vi "SetBaseCluster.vi"(7 "Actor":refnum<class "Actor.lvclass">, 11 "BaseCluster":T1) -> (5 "Actor":refnum<class "Actor.lvclass">)   [LabVIEW 2020, in "_Template.lvlib" / "{{Actor}}.lvlib" / "Actor.lvclass"]
uses:
  Actor.lvclass
  Actor.lvclass/Actor.ctl
  jettl/jettl/Actor/Actor.lvclass
  jettl/jettl/LifecycleEnum.ctl
  jettl/jettl/jettl.lvlib
  jettl/jettl/Message/Message.lvclass
  jettl/jettl/MessageSet.ctl
  jettl/jettl/MessagesCluster.ctl
  jettl/jettl/MessageCluster.ctl
  jettl/jettl/ActorTypeEnum.ctl
  jettl/jettl/ActorCluster.ctl
  jettl/jettl/ComponentActorClusterMap.ctl
  jettl/jettl/BaseCluster.ctl
  jettl/jettl/TellComponentMessageSetMap.ctl
  jettl/jettl/PostSetupCluster.ctl
  jettl/jettl/PreSetupCluster.ctl
  jettl/jettl/MainCluster.ctl
panel:
  # "This front panel should not be manipulated."
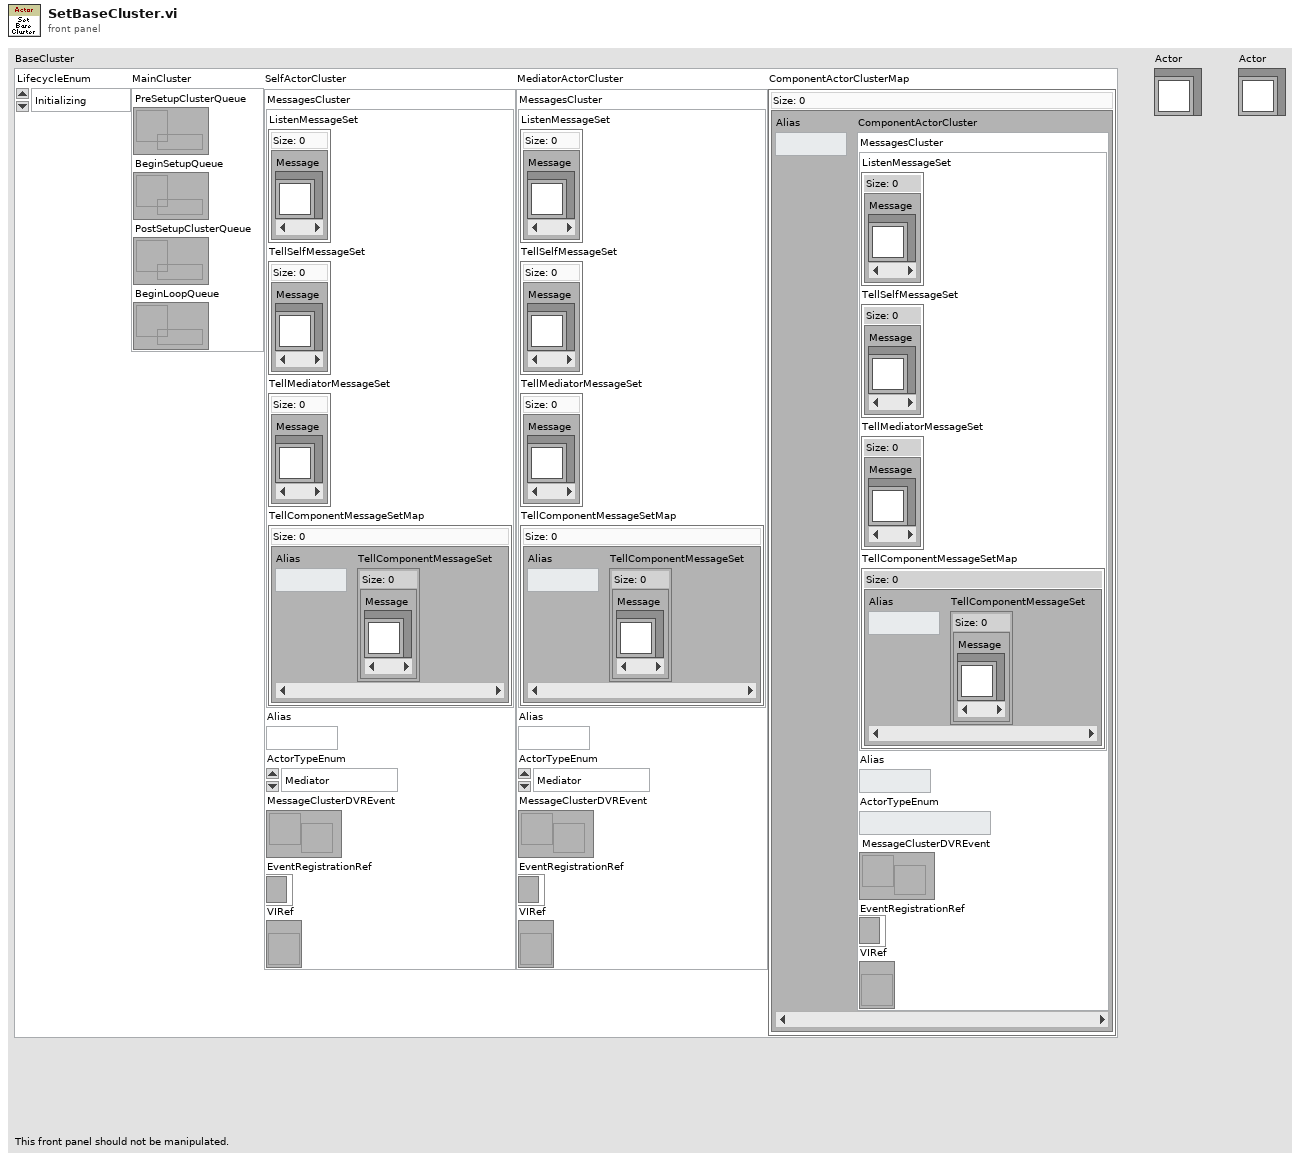
[diagram p1: front panel]
types:
  T1 = typedef "jettl.lvlib/BaseCluster.ctl" = cluster{"LifecycleEnum":T2, "MainCluster":T3, "SelfActorCluster":T4, "MediatorActorCluster":T4, "ComponentActorClusterMap":T9}
  T2 = typedef "jettl.lvlib/LifecycleEnum.ctl" = enum16{"Initializing", "SettingUp", "Starting", "Running", "Stopping", "TearingDown", "Terminated", "Abort"}
  T3 = typedef "jettl.lvlib/MainCluster.ctl" = cluster{"PreSetupClusterQueue":refnum<queue>, "BeginSetupQueue":refnum<queue>, "PostSetupClusterQueue":refnum<queue>, "BeginLoopQueue":refnum<queue>}
  T4 = typedef "jettl.lvlib/ActorCluster.ctl" = cluster{"MessagesCluster":T5, "Alias":string, "ActorTypeEnum":T8, "MessageClusterDVREvent":refnum<user-event>, "EventRegistrationRef":refnum<event-registration>, "VIRef":refnum<vi>}
  T5 = typedef "jettl.lvlib/MessagesCluster.ctl" = cluster{"ListenMessageSet":T6, "TellSelfMessageSet":T6, "TellMediatorMessageSet":T6, "TellComponentMessageSetMap":T7}
  T6 = typedef "jettl.lvlib/MessageSet.ctl" = set{refnum<class "Message.lvclass">}
  T7 = typedef "jettl.lvlib/TellComponentMessageSetMap.ctl" = map{string, T6}
  T8 = typedef "jettl.lvlib/ActorTypeEnum.ctl" = enum16{"Mediator", "Component"}
  T9 = typedef "jettl.lvlib/ComponentActorClusterMap.ctl" = map{string, T4}
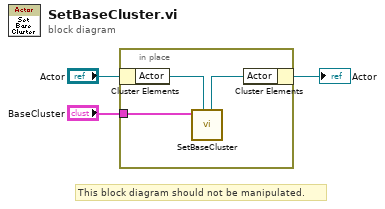
[diagram p0: block diagram]
diagram:
  # "This block diagram should not be manipulated."
  n1 = in-place {
    in-place-border: "BaseCluster" -> [w4]
    n2 = in-place-cluster #1("Actor") -> ("Actor"=w6:refnum<class "Actor.lvclass">)
    n3 = call-dynamic "SetBaseCluster.vi"("Actor"=w6, "BaseCluster"=w4) -> ("Actor"=w5:refnum<class "Actor.lvclass">)  [unwired: 9 in]
    n4 = in-place-cluster #1("Actor"=w5) -> (→"Actor":refnum<class "Actor.lvclass">)
  }
